vi "spec_GetGratings.vi"(8 "error in (no error)":errorcluster, 11 "LightField Automation in":refnum<class "LightField Automation.lvclass">) -> (0 "error out":errorcluster, 1 "Current Grating":string, 2 "Gratings":string[](array[string]), 3 "LightField Automation out":refnum<class "LightField Automation.lvclass">)   [LabVIEW 2018, in "LightField Automation.lvclass"]
uses:
  LightField Automation.lvclass
  C:/Users/xw9/Desktop/Turbulence program/SourceDistribution/PrincetonInstruments.LightFieldAddInSupportServices.dll
  PrincetonInstruments.LightFieldAddInSupportServices.dll
  LightField Automation.lvclass/LightField Automation.ctl
  C:/Users/xw9/Desktop/Turbulence program/SourceDistribution/PrincetonInstruments.LightFieldViewV3.dll
  PrincetonInstruments.LightFieldViewV3.dll
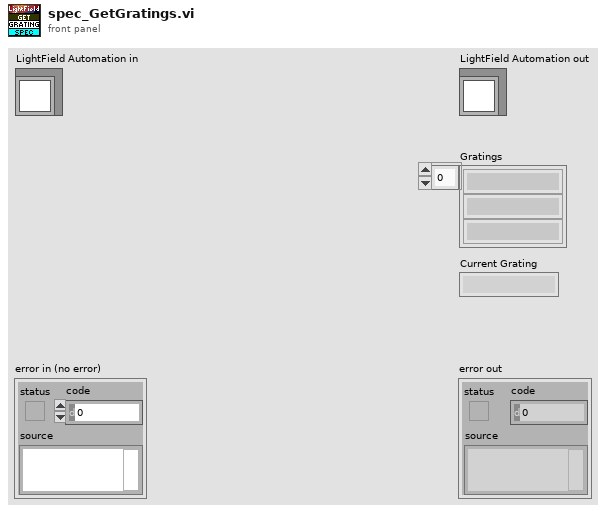
[diagram p1: front panel]
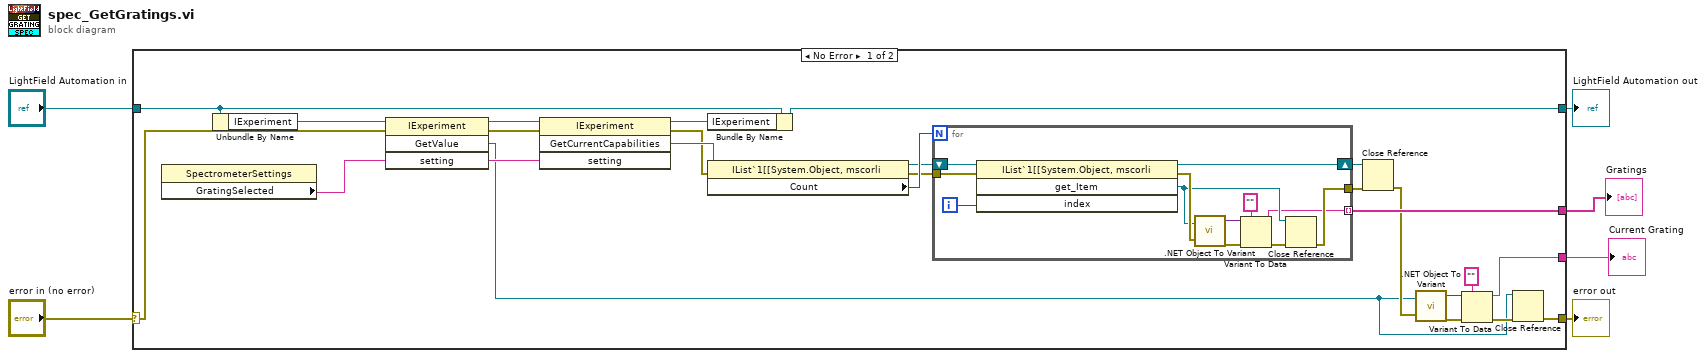
[diagram p0: block diagram]
diagram:
  n1 = case shown="No Error" "error in (no error)" {
    selector: "error in (no error)" -> [w16 w44]
    tunnel: [w8 w44] -> w5
    tunnel: [w29 w43] -> w3
    tunnel: "LightField Automation in" -> [w30 w43]
    tunnel: [w20 _] -> w2
    tunnel: [w10 _] -> w1
    frame No Error {
      n2 = property class="SpectrometerSettings"() -> ("GratingSelected"=w15:string)  [unwired: 2 in, 2 out]
      n3 = Unbundle By Name(w30) -> ("IExperiment"=w17:refnum<k24>)
      n4 = invoke class="IExperiment" method="GetValue"(reference=w17, error in=w16, "setting"=w15) -> (reference out=w19:refnum<k24>, error out=w18:errorcluster, "GetValue"=w7:refnum<k24>)  [unwired: 1 in, 1 out]
      n5 = invoke class="IExperiment" method="GetCurrentCapabilities"(reference=w19, error in=w18, "setting"=w15) -> (reference out=w28:refnum<k24>, error out=w26:errorcluster, "GetCurrentCapabilities"=w27:refnum<k24>)  [unwired: 1 in, 1 out]
      n6 = Bundle By Name(cluster=w30, "IExperiment"=w28) -> (w29:refnum<class "LightField Automation.lvclass">)
      n7 = property class="IList`1[[System.Object, mscorli"(reference=w27, error in=w26) -> (reference out=w24:refnum<k24>, error out=w23:errorcluster, "Count"=w25:i32)
      n8 = for {
        N: w25 -> [_]
        shift-right: [w40] -> w22
        shift-left: w24 -> [w42]
        tunnel: w23 -> [w41]
        tunnel: [w33] -> w21
        tunnel: [w32] -> w20 mode=indexing
        i -> [w31]
        n9 = invoke class="IList`1[[System.Object, mscorli" method="get_Item"(reference=w42, error in=w41, "index"=w31) -> (reference out=w40:refnum<k24>, error out=w36:errorcluster, "get_Item"=w34:refnum<k24>)  [unwired: 1 in, 1 out]
        n10 = call ".NET Object To Variant.vi"("error in (no error)"=w36, ".NET object"=w34) -> ("error out"=w39:errorcluster, "variant"=w37:variant)
        n11 = Variant To Data(error in=w39, type="" ("GratingSelected"), Variant=w37) -> (data=w32:string, error out=w35:errorcluster)
        n12 = Close Reference(reference=w34, error in (no error)=w35) -> (error out=w33:errorcluster)
      }
      n13 = Close Reference(reference=w22, error in (no error)=w21) -> (error out=w11:errorcluster)
      n14 = call ".NET Object To Variant.vi"("error in (no error)"=w11, ".NET object"=w7) -> ("error out"=w12:errorcluster, "variant"=w14:variant)
      n15 = Variant To Data(error in=w12, type="" ("GratingSelected"), Variant=w14) -> (data=w10:string, error out=w9:errorcluster)
      n16 = Close Reference(reference=w7, error in (no error)=w9) -> (error out=w8:errorcluster)
    }
    frame Error {
    }
  }
  "error out" <- w5
  "LightField Automation out" <- w3
  "Gratings" <- w2
  "Current Grating" <- w1
